vi "initiate.vi"(8 "error in (no error)":errorcluster, 11 "reference in":refnum<class "Project Panels.lvclass">) -> (0 "error out":errorcluster, 3 "reference out":refnum<class "Project Panels.lvclass">)   [LabVIEW 2016, in "Project Panels.lvclass"]
uses:
  Project Panels.lvclass
  SYS/Devices Controller_llb/Devices Controller.lvclass
  SYS/File Controller_llb/File Controller.lvclass
  SYS/Items Controller_llb/Items Controller.lvclass
  SYS/Notification Controller_class/Notification Controller.lvclass
  SYS/PartsTracking Controller_class/PartsTracking Controller.lvclass
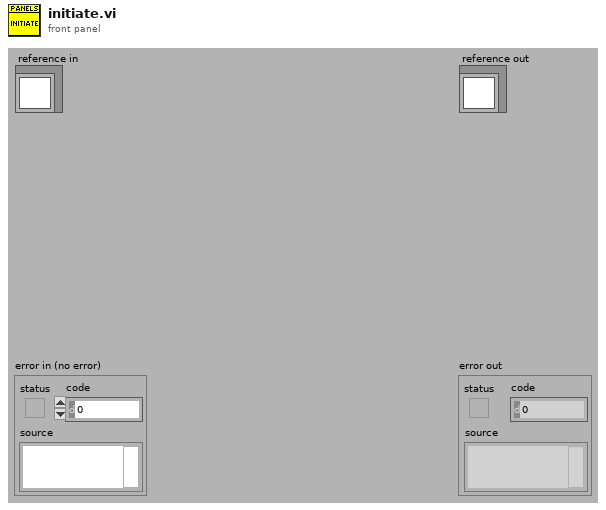
[diagram p1: front panel]
types:
  T1 = typedef "Project Panels.lvclass/ObjectAttributesRef.ctl" = refnum<data-value>
  T2 = typedef "Project Panels.lvclass/ObjectAttributes.ctl" = cluster{"MyAttribute":dbl, "device_controller_ref":refnum<class "Devices Controller.lvclass">, "file_controller_ref":refnum<class "File Controller.lvclass">, "item_controller_ref":refnum<class "Items Controller.lvclass">, "item_tables":cluster{"checkIN":string[][], "checkOUT":string[][], "storage":string[][]}, "quickbook_table":cluster{"notes":string[][]}, "notification_controller_ref":refnum<class "Notification Controller.lvclass">, "partstracking_controller_ref":refnum<class "PartsTracking Controller.lvclass">, "product_tables":cluster{"k4b2":string[][], "fitmate":string[][], "RMR":string[][], "CPET":string[][], "BP":string[][], "PP":string[][], "k5":string[][], "bb-pft":string[][]}, "rowsColour":u32[], "low_resolution?":bool, "run_python?":bool}
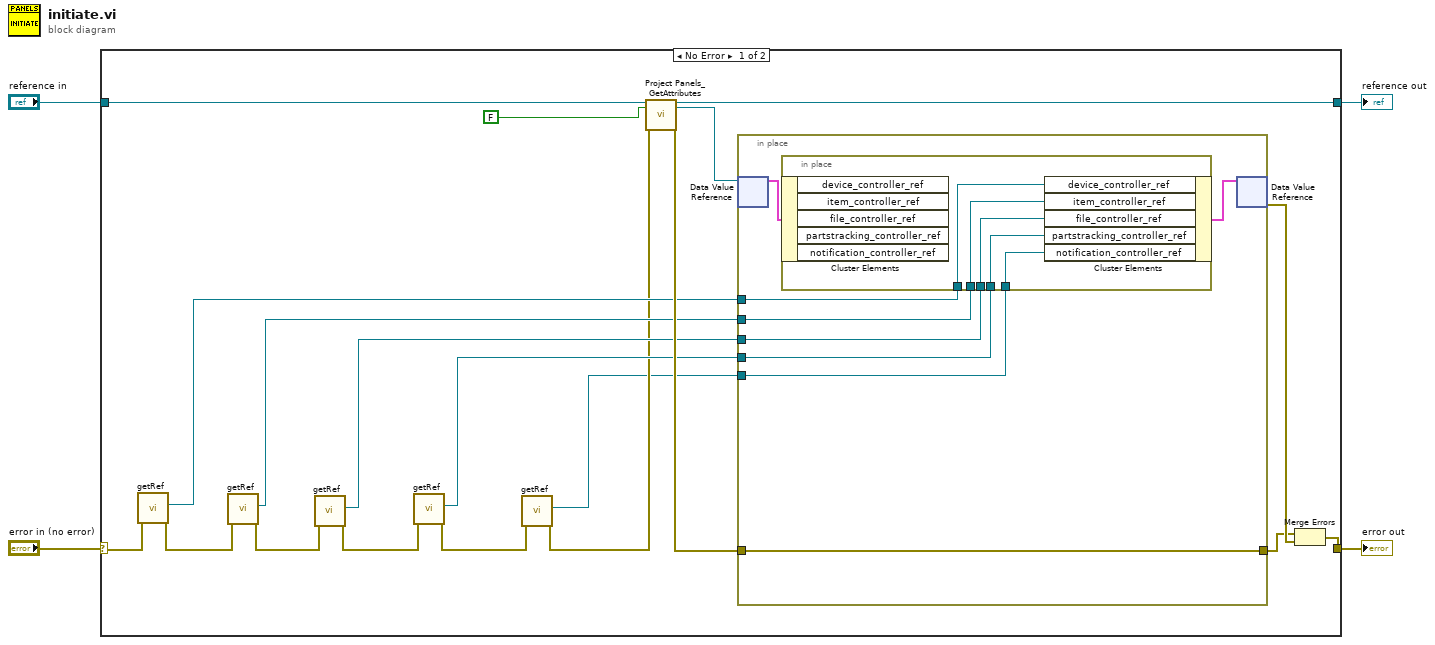
[diagram p0: block diagram]
diagram:
  n1 = case shown="No Error" "error in (no error)" {
    selector: "error in (no error)" -> [w15 w38]
    tunnel: [w23 w38] -> w3
    tunnel: [w17 w37] -> w1
    tunnel: "reference in" -> [w20 w37]
    frame No Error {
      n2 = call "getRef.vi"("error in (no error)"=w15) -> ("error out"=w14:errorcluster, "device_controller_ref"=w12:refnum<class "Devices Controller.lvclass">)  [unwired: 9 in]
      n3 = call "getRef.vi"("error in (no error)"=w14) -> ("error out"=w13:errorcluster, "items_controller_ref"=w11:refnum<class "Items Controller.lvclass">)  [unwired: 9 in]
      n4 = call "getRef.vi"("error in (no error)"=w13) -> ("error out"=w9:errorcluster, "File Controller_ref"=w10:refnum<class "File Controller.lvclass">)  [unwired: 9 in]
      n5 = call "getRef.vi"("error in (no error)"=w9) -> ("error out"=w7:errorcluster, "partstracking_controller_ref"=w8:refnum<class "PartsTracking Controller.lvclass">)  [unwired: 9 in]
      n6 = call "getRef.vi"("error in (no error)"=w7) -> ("error out"=w6:errorcluster, "notification_controller_ref"=w5:refnum<class "Notification Controller.lvclass">)  [unwired: 9 in]
      n7 = call "Project Panels_GetAttributes.vi"("reference in"=w20, "return data? (T)"=FALSE, "error in (no error)"=w6) -> ("reference out"=w17:refnum<class "Project Panels.lvclass">, "attributes ref"=w16:T1, "error out"=w18:errorcluster)  [unwired: 13 in, 1 out]
      n8 = in-place {
        in-place-border: w18 -> [w29]
        in-place-border: [w29] -> w21
        in-place-border: w12 -> [w28]
        in-place-border: w11 -> [w27]
        in-place-border: w10 -> [w26]
        in-place-border: w8 -> [w25]
        in-place-border: w5 -> [w24]
        n9 = in-place-dvr #1(w16) -> (w30:T2)  [unwired: 1 out]
        n10 = in-place {
          in-place-border: w28 -> [w36]
          in-place-border: w27 -> [w35]
          in-place-border: w26 -> [w34]
          in-place-border: w25 -> [w33]
          in-place-border: w24 -> [w32]
          n11 = in-place-cluster #2(w30) -> ()  [unwired: 5 out]
          n12 = in-place-cluster #2("device_controller_ref"=w36, "item_controller_ref"=w35, "file_controller_ref"=w34, "partstracking_controller_ref"=w33, "notification_controller_ref"=w32) -> (w31:T2)
        }
        n13 = in-place-dvr #1(w31) -> (w22:errorcluster)  [unwired: 1 out]
      }
      n14 = Merge Errors(w21, w22) -> (w23:errorcluster)
    }
    frame Error {
    }
  }
  "error out" <- w3
  "reference out" <- w1
